vi "3D Intensity plot.vi"() -> ()   [LabVIEW 2015]
panel:
  out "Array":dbl[][](array[numeric])
  out "Intensity Graph":dbl[][](graph)
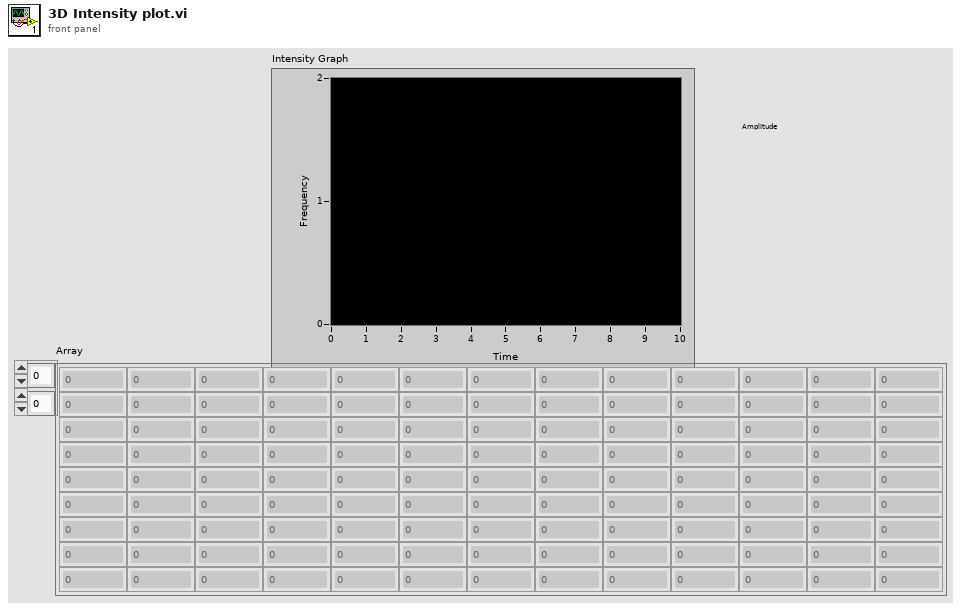
[diagram p1: front panel]
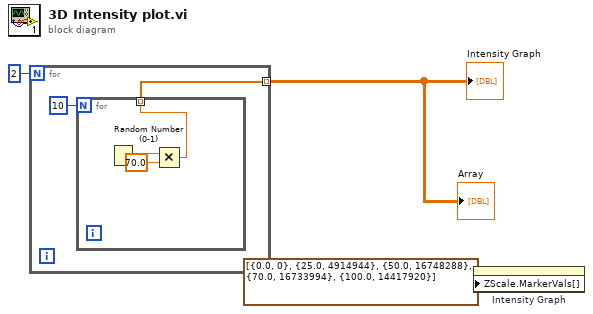
[diagram p0: block diagram]
diagram:
  n1 = for {
    N: 2 -> [_]
    tunnel: [w4] -> w2 mode=indexing
    n2 = for {
      N: 10 -> [_]
      tunnel: [w6] -> w4 mode=indexing
      n3 = Random Number (0-1)() -> (number: 0 to 1=w8:dbl)
      n4 = Multiply(x=w8, y=70.0) -> (x*y=w6:dbl)
    }
  }
  "Intensity Graph" <- w2
  "Array" <- w2
  n5 = property on="Intensity Graph" class="IntGraph (strict)"("ZScale.MarkerVals[]"=cluster{dbl, u32}[] [{0.0, 0}, {25.0, 4914944}, {50.0, 16748288}, {70.0, 16733994}, {100.0, 14417920}] ("Z Scale.Marker Values[]")) -> ()  [unwired: 2 in, 2 out]
